vi "Main.vi"() -> ()   [LabVIEW 2021]
uses:
  <vilib>/ptbypt/NI_PtbyPt.lvlib
panel:
  out "Cluster":cluster{"Number of tries":dbl, "Tries":dbl[]}
  out "Output":string
  in  "Guess":dbl
  out "String":string
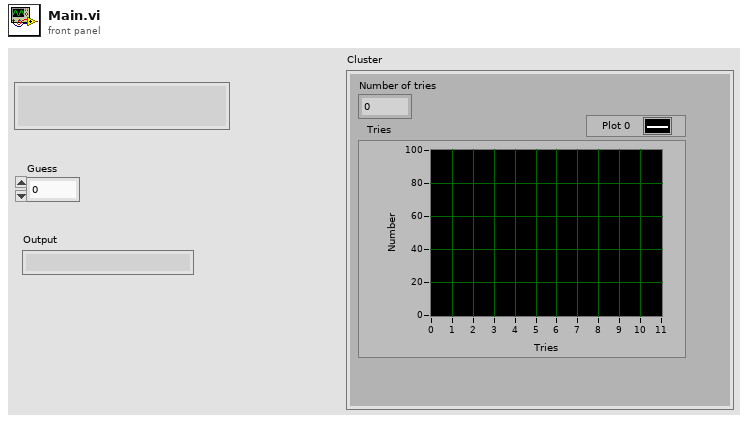
[diagram p1: front panel]
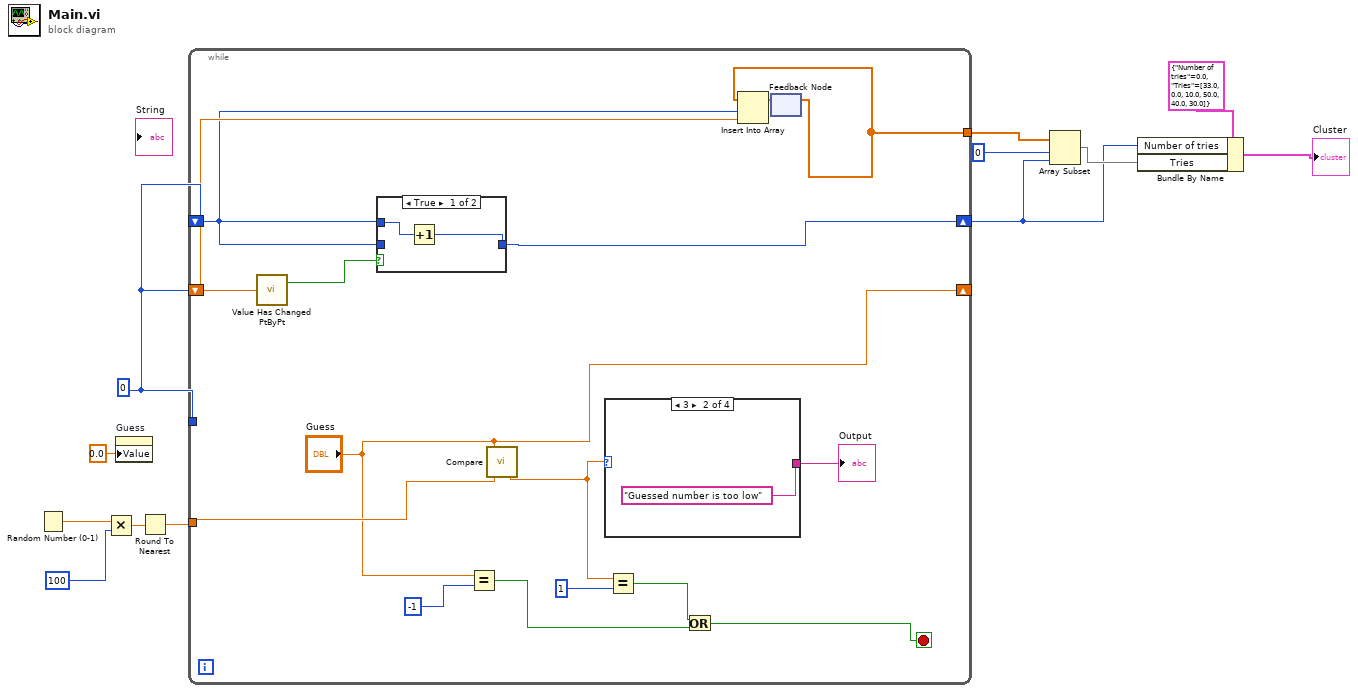
[diagram p0: block diagram]
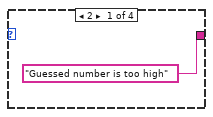
[diagram p3: hidden frame]
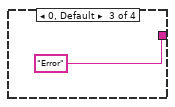
[diagram p4: hidden frame]
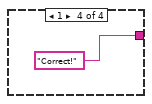
[diagram p5: hidden frame]
diagram:
  w8 = 0
  n1 = Random Number (0-1)() -> (number: 0 to 1=w11:dbl)
  n2 = Multiply(x=w11, y=100) -> (x*y=w10:dbl)
  n3 = property on="Guess" class="DigNum (strict)"("Value"=0.0 ("Guess")) -> ()  [unwired: 2 in, 2 out]
  n4 = Round To Nearest(number=w10) -> (nearest integer value=w9:dbl)
  n5 = while {
    tunnel: w9 -> [w25]
    tunnel: w8 -> [_]
    shift-right: ["Guess"] -> _
    shift-left: w8 -> [w16]
    shift-right: [w17] -> w1
    shift-left: w8 -> [w14]
    tunnel: [w13] -> w6
    stop <- w24 stop-if-true
    n6 = call <vilib>:"Value Has Changed PtByPt.vi"("input data point"=w16) -> ("has changed"=w18:bool)  [unwired: 1 in, 1 out]
    n7 = case shown="True" w18 {
      tunnel: [w29 w30] -> w17
      tunnel: w14 -> [w28 _]
      tunnel: w14 -> [_ w30]
      frame True {
        n8 = Increment(x=w28) -> (x+1=w29:i32)
      }
      frame False {
      }
    }
    n9 = Equal?(x="Guess", y=-1) -> (x = y?=w21:bool)
    n10 = call "Compare.vi"("RandomNumber"=w25, "Guessed number"="Guess") -> ("Output"=w20:dbl)
    n11 = case shown="3" w20 {
      tunnel: ["Guessed number is too high" "Guessed number is too low" "Error" "Correct!"] -> w27
      frame 2 {
      }
      frame 3 {
      }
      frame 0, Default {
      }
      frame 1 {
      }
    }
    "Output" <- w27
    n12 = Equal?(x=w20, y=1) -> (x = y?=w23:bool)
    n13 = Or(x=w23, y=w21) -> (x .or. y?=w24:bool)
    n14 = feedback #1() -> (w13:dbl[])  [unwired: 1 in]
    n15 = Insert Into Array(array=w13, index=w14, new element=w16) -> (w15:dbl[])
    n16 = feedback-in #1(w15) -> ()
  }
  n17 = Array Subset(array=w6, index=0, length=w1) -> (w3:dbl[])
  n18 = Bundle By Name(cluster=cluster{"Number of tries":dbl, "Tries":dbl[]} {"Number of tries"=0.0, "Tries"=[33.0, 0.0, 10.0, 50.0, 40.0, 30.0]} ("Cluster"), "Number of tries"=w1, "Tries"=w3) -> (→"Cluster":cluster{"Number of tries":dbl, "Tries":dbl[]})
